vi "WinCI Check In.vi"(6 "keep checked out? (F)":bool, 7 "advanced options":variant, 8 "error in (no error)":errorcluster, 9 "comment":string, 10 "files":path[](array[path]), 11 "source control reference in":T1) -> (0 "error out":errorcluster, 1 "dialog box cancelled?":bool, 2 "status message":string, 3 "source control reference out":T1)   [LabVIEW 2017, in "NI_SCC_WinCI.lvlib"]
uses:
  <vilib>/SourceControl/Providers/WinCI/NI_SCC_WinCI.lvlib
  <vilib>/SourceControl/sccapi/SCCAPI Refnum.ctl
  <vilib>/SourceControl/support/SCCSup Message Strings GLBL.vi
  <vilib>/SourceControl/sccapi/NI_SCC.lvlib
panel:
  out "result":i32
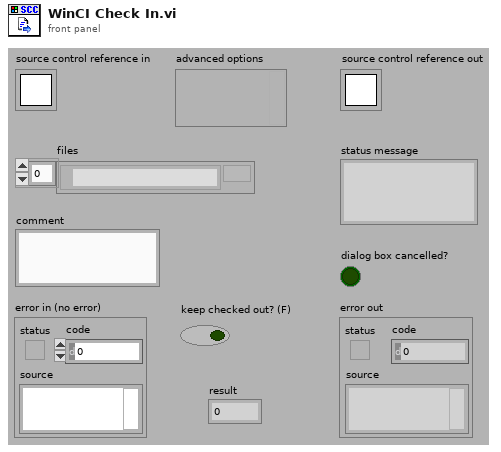
[diagram p1: front panel]
types:
  T1 = typedef "NI_SCC.lvlib/SCCAPI Refnum.ctl" = refnum<k1>
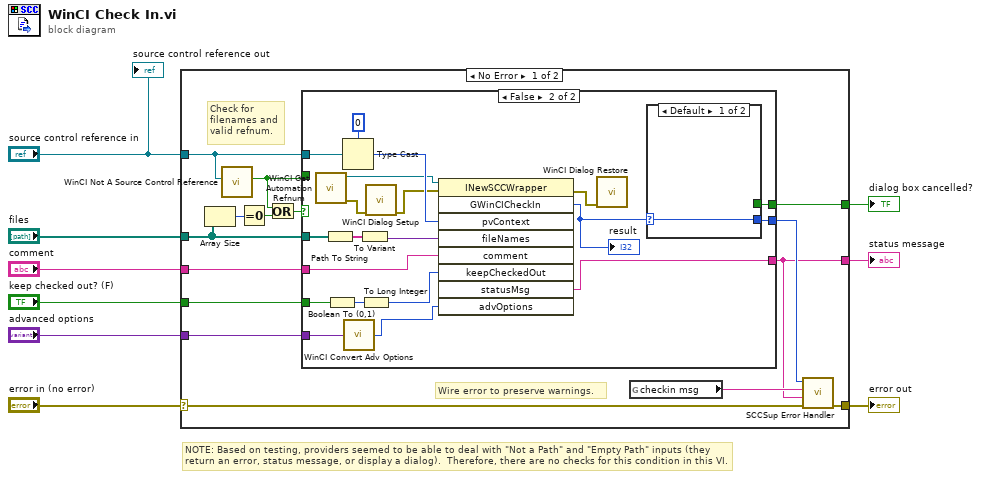
[diagram p0: block diagram]
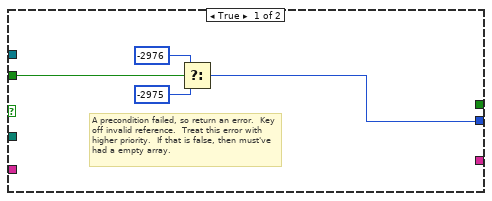
[diagram p2: hidden frame]
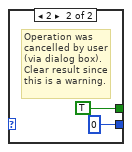
[diagram p3: hidden frame]
diagram:
  # "NOTE: Based on testing, providers seemed to be able to deal with \"Not a Path\" and \"Empty Path\" inputs (they return an error, status message, or display a dialog).  Therefore, there are no checks for this condition in this VI."
  n1 = case shown="No Error" "error in (no error)" {
    selector: "error in (no error)" -> [w14 w52]
    tunnel: [w22 w52] -> w8
    tunnel: "source control reference in" -> [w10 _]
    tunnel: [w19 _] -> w6
    tunnel: "files" -> [w16 _]
    tunnel: "comment" -> [w24 _]
    tunnel: "keep checked out? (F)" -> [w23 _]
    tunnel: [w13 _] -> w2
    tunnel: "advanced options" -> [w12 _]
    frame No Error {
      # "Wire error to preserve warnings."
      # "Check for filenames and valid refnum."
      n2 = Array Size(array=w16) -> (size(s)=w18:i32)
      n3 = call <vilib>:"WinCI Not A Source Control Reference.vi"("source control reference in"=w10) -> ("not a source control reference?"=w11:bool)  [unwired: 1 in, 9 out]
      n4 = Equal To 0?(x=w18) -> (x = 0?=w17:bool)
      n5 = Or(x=w11, y=w17) -> (x .or. y?=w15:bool)
      n6 = case shown="False" w15 {
        tunnel: w10 -> [_ w48]
        tunnel: [_ w34] -> w19
        tunnel: w16 -> [_ w46]
        tunnel: w24 -> [_ w37]
        tunnel: w23 -> [_ w44]
        tunnel: [w25 w43] -> w21
        tunnel: w11 -> [w26 _]
        tunnel: [_ w42] -> w13
        tunnel: w12 -> [_ w41]
        frame True {
          # "A precondition failed, so return an error.  Key off invalid reference.  Treat this error with higher priority.  If that is false, then must've had a empty array."
          n7 = Select(t=-2976 ("result"), s=w26, f=-2975 ("result")) -> (s? t:f=w25:i32)
        }
        frame False {
          n8 = call <vilib>:"WinCI Get Automation Refnum.vi"() -> ("error out"=w31:errorcluster, "automation refnum"=w32:refnum<k7>)  [unwired: 10 out]
          n9 = Path To String(path=w46) -> (string=w40:string[])
          n10 = Boolean To (0,1)(Boolean=w44) -> (0, 1=w45:i16)
          n11 = Type Cast(type=u32 0, x=w48) -> (*(type *) &x=w35:u32)
          n12 = call <vilib>:"WinCI Convert Adv Options.vi"("advanced options"=w41) -> ("command options"=w39:u32)  [unwired: 4 out]
          n13 = To Variant(anything=w40) -> (Variant=w36:variant)
          n14 = To Long Integer(number=w45) -> (32bit integer=w38:i32)
          n15 = call <vilib>:"WinCI Dialog Setup.vi"("error in"=w31) -> ("error out"=w30:errorcluster)  [unwired: 10 out]
          n16 = invoke class="INewSCCWrapper" method="GWinCICheckIn"(reference=w32, error in=w30, "pvContext"=w35, "fileNames"=w36, "comment"=w37, "keepCheckedOut"=w38, "advOptions"=w39) -> (error out=w29:errorcluster, "GWinCICheckIn"=w33:i32, "statusMsg"=w34:string)  [unwired: 2 in, 6 out]
          "result" <- w33
          n17 = call <vilib>:"WinCI Dialog Restore.vi"("error in"=w29) -> ()  [unwired: 11 out]
          n18 = case shown="Default" w33 {
            selector: w33 -> [w49 _]
            tunnel: [w49 0 ("result")] -> w43
            tunnel: [_ TRUE] -> w42
            frame Default {
            }
            frame 2 {
              # "Operation was cancelled by user (via dialog box).  Clear result since this is a warning."
            }
          }
        }
      }
      n19 = global read "SCCSup Message Strings GLBL.vi" "checkin msg"() -> (w20:string)
      n20 = call <vilib>:"SCCSup Error Handler.vi"("error in (no error)"=w14, "additional message"=w19, "operation message"=w20, "scc error code"=w21) -> ("error out"=w22:errorcluster)  [unwired: 7 out]
    }
    frame Error {
    }
  }
  "error out" <- w8
  "status message" <- w6
  "dialog box cancelled?" <- w2
  "source control reference out" <- "source control reference in"
